vi "test Create New at Existing Path.vi"(8 "error in (no error)":errorcluster, 11 "TestCase in":refnum<class "Configuration Tests.lvclass">) -> (0 "error out":errorcluster, 3 "TestCase out":refnum<class "Configuration Tests.lvclass">)   [LabVIEW 2017, in "Configuration Tests.lvclass"]
uses:
  Configuration Tests.lvclass
  <vilib>/addons/_JKI Toolkits/VI Tester/TestCase.llb/TestCase.lvclass
  Configuration/Configuration Session.lvclass
  C:/Program Files (x86)/National Instruments/LabVIEW 2017/vi.lib/addons/_JKI Toolkits/VI Tester/TestCase.llb/TestCase.lvclass
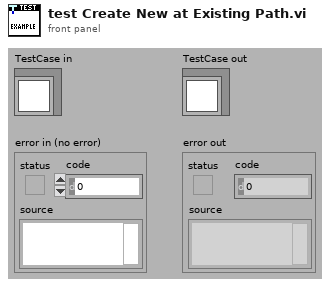
[diagram p1: front panel]
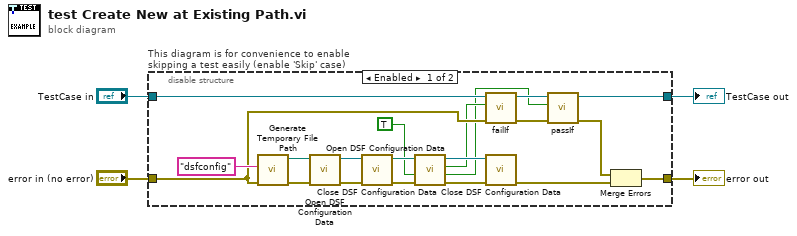
[diagram p0: block diagram]
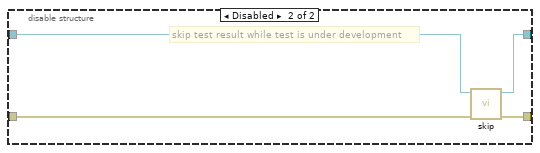
[diagram p2: hidden frame]
diagram:
  n1 = disable-structure "This diagram is for convenience to enable skipping a test easily (enable 'Skip' case)" shown="Enabled" {
    disable-tunnel: "TestCase in" -> [w21 w28]
    disable-tunnel: [w7 w26] -> w1
    disable-tunnel: [w19 w27] -> w3
    disable-tunnel: "error in (no error)" -> [w20 w25]
    frame Enabled {
      n2 = call <vilib>:"Generate Temporary File Path.vi"("error in (no error)"=w20, "Temporary File Extension (tmp)"="dsfconfig") -> ("error out"=w23:errorcluster, "Unique Temporary File Path"=w24:path)  [unwired: 8 in]
      n3 = call "Open DSF Configuration Data.vi"("error in (no error)"=w23, "dsf configuration file path"=w24) -> ("error out"=w18:errorcluster, "Configuration Session"=w16:refnum<class "Configuration Session.lvclass">)  [unwired: 5 in, 3 out]
      n4 = call "Close DSF Configuration Data.vi"("error in (no error)"=w18, "Configuration Session"=w16) -> ("error out"=w17:errorcluster, "file path"=w15:path)  [unwired: 8 in]
      n5 = call "Open DSF Configuration Data.vi"("error in (no error)"=w17, "replace if found? (F)"=TRUE, "dsf configuration file path"=w15) -> ("error out"=w13:errorcluster, "file replaced?"=w6:bool, "file created?"=w10:bool, "Configuration Session"=w14:refnum<class "Configuration Session.lvclass">)  [unwired: 4 in, 1 out]
      n6 = call-dynamic "failIf.vi"("error in (no error)"=w20, "fail"=w10, "TestCase in"=w21) -> ("error out"=w11:errorcluster, "TestCase out"=w8:refnum<class "Configuration Tests.lvclass">)  [unwired: 7 in]
      n7 = call "Close DSF Configuration Data.vi"("error in (no error)"=w13, "Configuration Session"=w14) -> ("error out"=w12:errorcluster)  [unwired: 8 in, 1 out]
      n8 = call-dynamic "passIf.vi"("error in (no error)"=w11, "pass"=w6, "TestCase in"=w8) -> ("error out"=w9:errorcluster, "TestCase out"=w7:refnum<class "Configuration Tests.lvclass">)  [unwired: 7 in]
      n9 = Merge Errors(w9, w12) -> (w19:errorcluster)
    }
    frame Disabled {
      # "skip test result while test is under development"
      n10 = call <vilib>:"skip.vi"("error in (no error)"=w25, "TestCase in"=w28) -> ("error out"=w27:errorcluster, "TestCase out"=w26:refnum<class "Configuration Tests.lvclass">)  [unwired: 8 in]
    }
  }
  "error out" <- w3
  "TestCase out" <- w1
